vi "Execute.vi"(8 "error in (no error)":errorcluster, 10 "ObserverRegistry in":refnum<class "ObserverRegistry.lvclass">, 11 "ObserverRegistryCommand":refnum<class "ObserverRegistryCommand.lvclass">) -> (0 "error out":errorcluster, 2 "ObserverRegistry out":refnum<class "ObserverRegistry.lvclass">, 3 "Message":refnum<class "MSG.lvclass">)   [LabVIEW 2011, in "Messenging.lvlib" / "ObserverRegistryCommand.lvclass"]
uses:
  ObserverRegistryCommand.lvclass
  ObserverRegistry.lvclass
  Interprocess Messenger/TextVarientMessage/MSG.lvclass
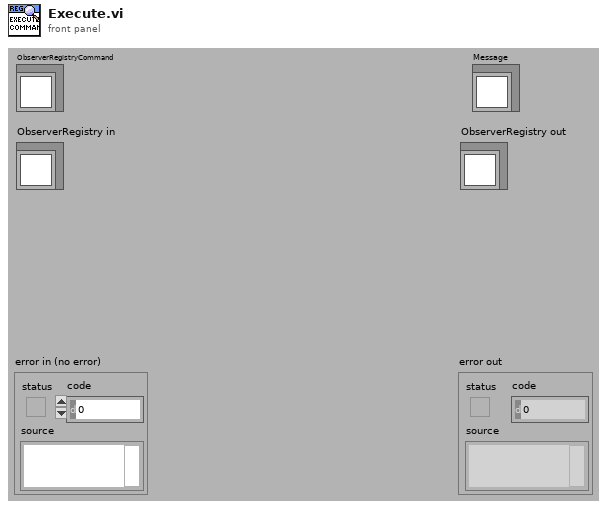
[diagram p1: front panel]
types:
  T1 = typedef "Messenging.lvlib/ObserverRegistry.lvclass/ObserverRegistryData.ctl" = cluster{"Observer of Errors":refnum<class "Observer.lvclass">, "Observer of All":refnum<class "Observer.lvclass">, "Event Registry":variant}
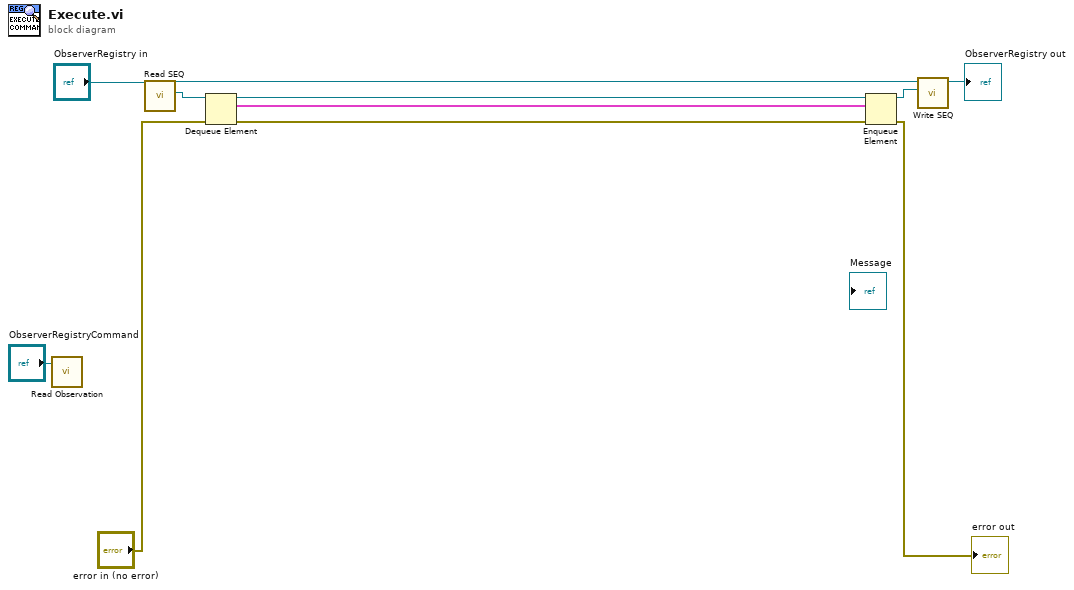
[diagram p0: block diagram]
diagram:
  n1 = call "Read Observation.vi"("ObserverRegistryCommand.lvclass in"="ObserverRegistryCommand") -> ()  [unwired: 1 in, 10 out]
  n2 = call "Read SEQ.vi"("ObserverRegistry.lvclass in"="ObserverRegistry in") -> ("SEQ"=w7:refnum<queue>, "ObserverRegistry.lvclass out"=w5:refnum<class "ObserverRegistry.lvclass">)  [unwired: 1 in, 8 out]
  n3 = Dequeue Element(queue=w7, error in (no error)="error in (no error)") -> (queue out=w11:refnum<queue>, element=w1:T1, error out=w2:errorcluster)  [unwired: 2 out]
  n4 = Enqueue Element(queue=w11, element=w1, error in (no error)=w2) -> (queue out=w4:refnum<queue>, error out=→"error out":errorcluster)  [unwired: 2 out]
  n5 = call "Write SEQ.vi"("SEQ"=w4, "ObserverRegistry.lvclass in"=w5) -> ("ObserverRegistry.lvclass out"=→"ObserverRegistry out":refnum<class "ObserverRegistry.lvclass">)  [unwired: 1 in, 8 out]
